vi "add_twist.vi"(4 "Twist":T1, 5 "msg in":string) -> (2 "msg out":string)   [LabVIEW 2012]
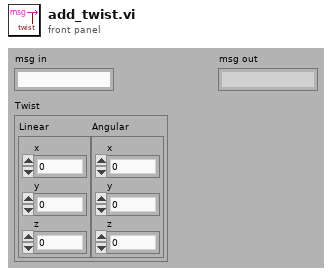
[diagram p1: front panel]
types:
  T1 = cluster{"Linear":cluster{"x":dbl, "y":dbl, "z":dbl}, "Angular":cluster{"x":dbl, "y":dbl, "z":dbl}}
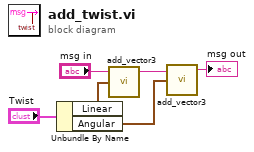
[diagram p0: block diagram]
diagram:
  n1 = Unbundle By Name("Twist") -> ("Linear"=w4:cluster{"x":dbl, "y":dbl, "z":dbl}, "Angular"=w3:cluster{"x":dbl, "y":dbl, "z":dbl})
  n2 = call <userlib>:"add_vector3.vi"("Vector3"=w4, "msg in"="msg in") -> ("msg out"=w6:string)  [unwired: 3 in]
  n3 = call <userlib>:"add_vector3.vi"("Vector3"=w3, "msg in"=w6) -> ("msg out"=→"msg out":string)  [unwired: 3 in]
